vi "Liquid Lens Process.vi"(8 "error in":errorcluster caption="error out") -> (0 "error out":errorcluster)   [LabVIEW 2015, in "Debug.lvlib"]
uses:
  Debug.lvlib
  Support/Liquid Lens Process State.ctl
  <vilib>/Instr/_visa.llb/VISA Configure Serial Port (Instr).vi
  Sub VIs/Serial/Serial.lvlib
panel:
  in  "停止按钮":bool
  in  "Value":i32
  in  "输出电压":i32(slide) scale=0.0..1024.0
  # "Liquid Lens Process"
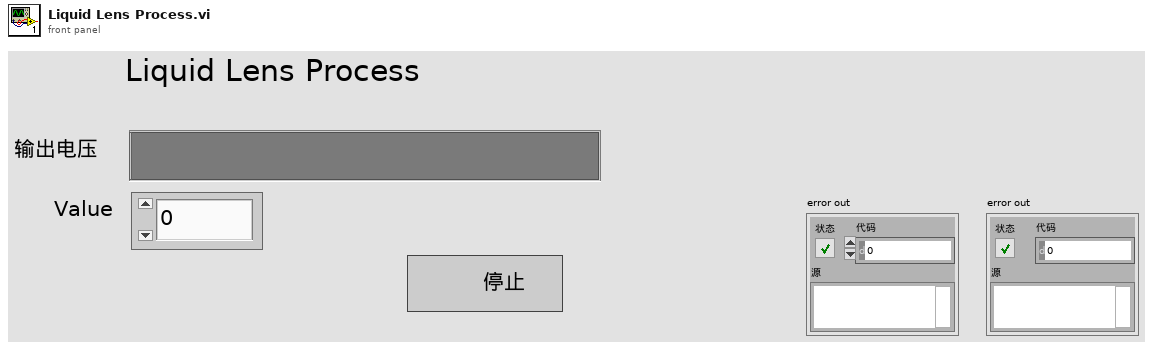
[diagram p1: front panel]
types:
  T1 = typedef "Debug.lvlib/Liquid Lens Process State.ctl" = enum16{"Initialize", "Update Settings", "Send Message", "Receive Message", "Wait For Event", "Exit"}
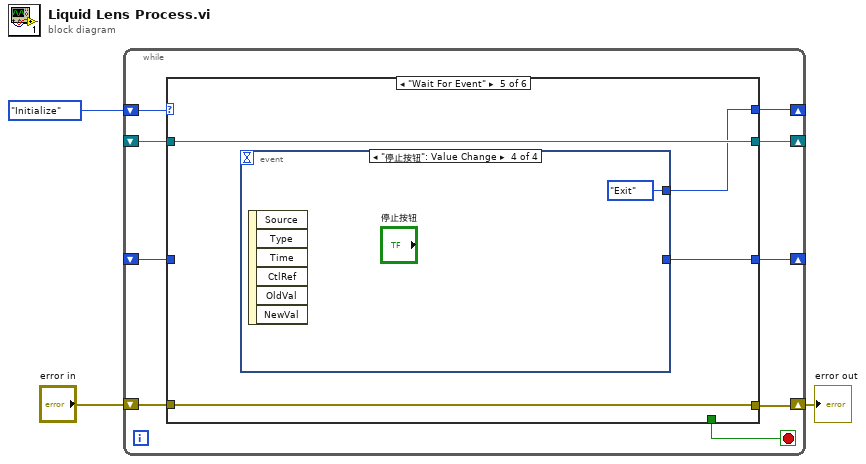
[diagram p0: block diagram]
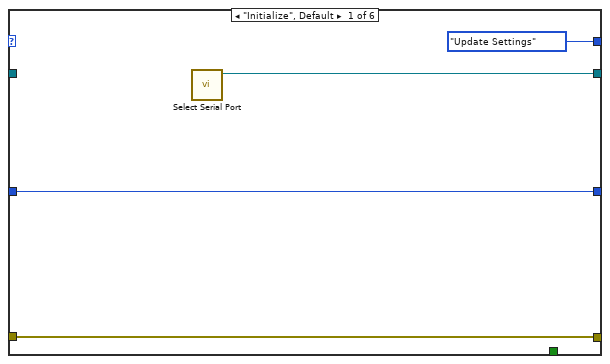
[diagram p2: hidden frame]
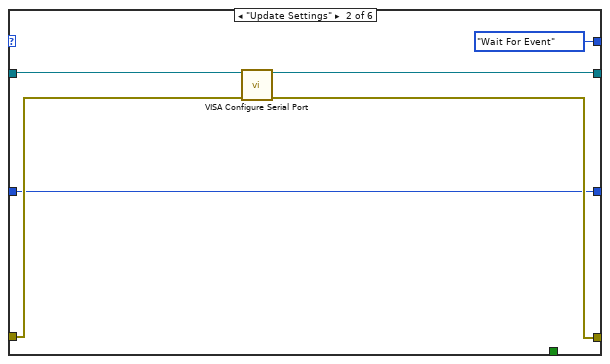
[diagram p3: hidden frame]
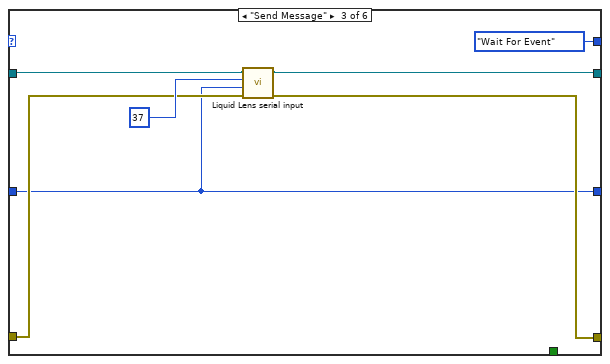
[diagram p4: hidden frame]
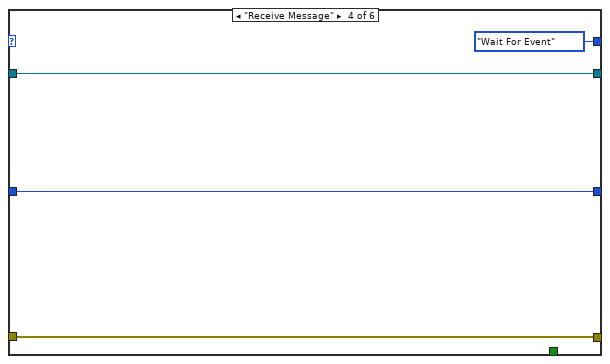
[diagram p5: hidden frame]
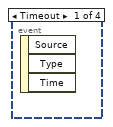
[diagram p6: hidden frame]
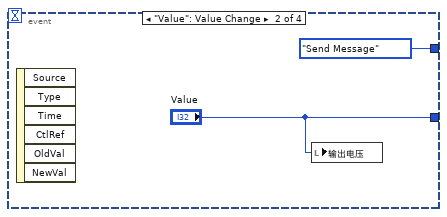
[diagram p7: hidden frame]
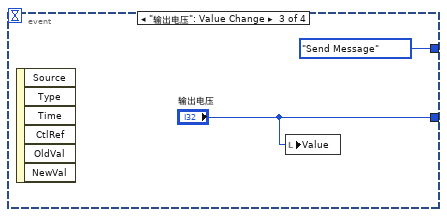
[diagram p8: hidden frame]
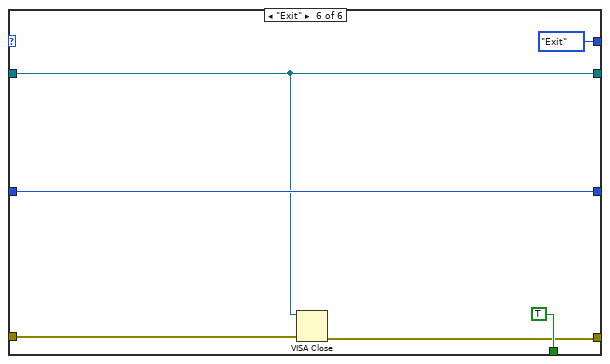
[diagram p9: hidden frame]
diagram:
  n1 = while {
    shift-right: [w11] -> _
    shift-left: _ -> [w10]
    shift-right: [w9] -> _
    shift-left: Liquid_Lens_Process_State."Initialize" ("Calculation Distance State") -> [w12]
    shift-right: [w8] -> w1
    shift-left: "error in" -> [w7]
    shift-right: [w6] -> _
    shift-left: _ -> [w5]
    stop <- w4 stop-if-true
    n2 = case shown="\"Wait For Event\"" w12 {
      tunnel: [w16 w21 w27 w32 w37 w43] -> w11
      tunnel: w10 -> [_ w22 w28 w32 w37 w43]
      tunnel: [Liquid_Lens_Process_State."Update Settings" ("Calculation Distance State") Liquid_Lens_Process_State."Wait For Event" ("Calculation Distance State") Liquid_Lens_Process_State."Wait For Event" ("Calculation Distance State") Liquid_Lens_Process_State."Wait For Event" ("Calculation Distance State") w35 Liquid_Lens_Process_State."Exit" ("Calculation Distance State")] -> w9
      tunnel: [w14 w18 w25 w31 w36 w44] -> w8
      tunnel: w7 -> [w14 w19 w24 w31 w36 w45]
      tunnel: [w13 w17 w23 w30 w34 w47] -> w6
      tunnel: w5 -> [w13 w17 w23 w30 _ w47]
      tunnel: [_ _ _ _ _ TRUE] -> w4
      frame "Initialize", Default {
        n3 = call "Select Serial Port.vi"() -> ("VISA资源名称 2"=w16:refnum<visa-resource-name>)  [unwired: 11 in]
      }
      frame "Update Settings" {
        n4 = call-poly "VISA Configure Serial Port"("VISA resource name"=w22, "error in (no error)"=w19) -> ("VISA resource name out"=w21:refnum<visa-resource-name>, "error out"=w18:errorcluster)  [unwired: 12 in]
      }
      frame "Send Message" {
        n5 = call "Liquid Lens serial input.vi"("错误输入（无错误）"=w24, "parameter"=w23, "item"=u8 37, "VISA资源名称"=w28) -> ("错误输出"=w25:errorcluster, "VISA资源名称输出"=w27:refnum<visa-resource-name>)  [unwired: 6 in]
      }
      frame "Receive Message" {
      }
      frame "Wait For Event" {
        n6 = event shown="[3] \"停止按钮\": Value Change" {
          selector: _ -> [_ _ _ _]
          dyn-events: _ -> [_ _ _ _]
          timeout: _ -> [_ _ _ _]
          tunnel: [_ Liquid_Lens_Process_State."Send Message" ("Calculation Distance State") Liquid_Lens_Process_State."Send Message" ("Calculation Distance State") Liquid_Lens_Process_State."Exit" ("Calculation Distance State")] -> w35
          tunnel: [_ "Value" "输出电压" _] -> w34
          event Timeout {
            n7 = event-data() -> ()  [unwired: 1 in, 3 out]
          }
          event "Value": Value Change {
            n8 = event-data() -> ()  [unwired: 1 in, 6 out]
            n9 = local write "输出电压"("Value") -> ()
          }
          event "输出电压": Value Change {
            n10 = event-data() -> ()  [unwired: 1 in, 6 out]
            n11 = local write "Value"("输出电压") -> ()
          }
          event "停止按钮": Value Change {
            n12 = event-data() -> ()  [unwired: 1 in, 6 out]
          }
        }
      }
      frame "Exit" {
        n13 = VISA Close(VISA resource name=w43, error in (no error)=w45) -> (error out=w44:errorcluster)
      }
    }
  }
  "error out" <- w1
